vi "Last Ack Created.vi"(10 "jettl":refnum<class "jettl.lvclass">) -> (2 "Msg Strategy":refnum<class "Msg Strategy.lvclass">)   [LabVIEW 2021, in "jettl.lvlib" / "Last Ack Created Msg Strategy.lvlib"]
uses:
  Last Ack Created Msg Strategy.lvlib
  Msg Strategy/Msg Strategy.lvclass
  jettl/jettl.lvclass
  Last Ack Created Msg Strategy/Last Ack Created Msg Strategy.lvclass
  C:/git/jettl/jettl/jettl/Msg Strategy/Msg Strategy.lvclass
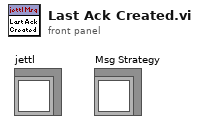
[diagram p1: front panel]
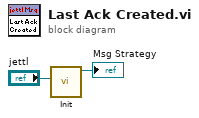
[diagram p0: block diagram]
diagram:
  n1 = call "Init.vi"("jettl"="jettl") -> ("Last Ack Created Msg Strategy out"=→"Msg Strategy":refnum<class "Last Ack Created Msg Strategy.lvclass">)  [unwired: 10 in]
